vi "FRCts20_Backend_TestReturnData.vi"() -> ()   [LabVIEW 2014, in "FRCts20_Backend_TestCode.lvlib"]
uses:
  FRCts20_Backend_TestCode.lvlib
  FRCts20_Backend_Engine.lvlib
  FRCts20_Backend_DequeueDataOperations.ctl
panel:
  out "Key":string
  out "Message Value":string
  out "Message Name":string
  out "error out":errorcluster
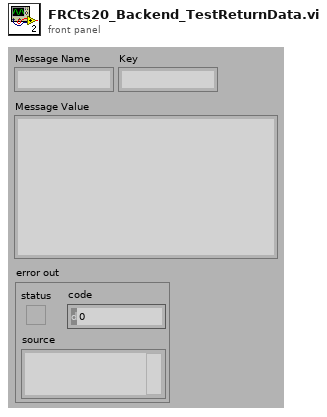
[diagram p1: front panel]
types:
  T1 = typedef "FRCts20_Backend_Engine.lvlib/FRCts20_Backend_DequeueDataOperations.ctl" = enum16{"Initialize", "DequeueDataReturn", "GetQueues"}
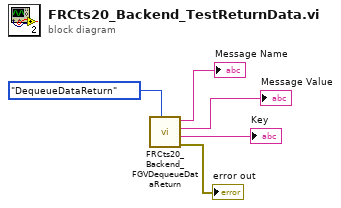
[diagram p0: block diagram]
diagram:
  n1 = call "FRCts20_Backend_FGVDequeueDataReturn.vi"("Operation"=FRCts20_Backend_DequeueDataOperations."DequeueDataReturn") -> ("error out"=→"error out":errorcluster, "Key"=→"Key":string, "Message Value"=→"Message Value":string, "Message Name"=→"Message Name":string)  [unwired: 6 in, 1 out]
